vi "Comparison of BLAS and linear algebra VIs.vi"() -> ()   [LabVIEW 2023]
doc: "This example compares the use of the Basic Linear Algebra Subroutines (BLAS) VIs with the use of the Linear Algebra VIs."
uses:
  <vilib>/Analysis/BLAS.llb/LV_Transpose.ctl
  <vilib>/Analysis/baseanly.llb/Real Dot Product.vi
  <vilib>/Analysis/7linalg.llb/Complex Conjugate Transpose Matrix.vi
  <vilib>/Analysis/baseanly.llb/Complex A x Vector.vi
  <vilib>/Analysis/7linalg.llb/Real Transpose Matrix.vi
  <vilib>/Analysis/baseanly.llb/Real A x B.vi
  <vilib>/Analysis/2dsp.llb/Decimate (continuous, DBL).vi
  <vilib>/Analysis/BLAS.llb/zgemv - General Matrix-Vector Product (CDB).vi
  <vilib>/Analysis/Matrix/Numeric/Multiply/Multiply - R,RM.vi
  <vilib>/Analysis/Matrix/Numeric/Add/Add - RM,RM.vi
  <vilib>/Analysis/BLAS.llb/dgemm - General Matrix-Matrix Product (DBL).vi
  <vilib>/Analysis/NI_AALBLAS.lvlib
  <vilib>/Analysis/NI_AALBase.lvlib
  <vilib>/Analysis/Matrix/NI_Matrix.lvlib
  <vilib>/Analysis/NI_AALPro.lvlib
panel:
  in  "Tab Control":T1(tab)
  out "BLAS result":dbl
  in  "y":dbl[](array[numeric])=[4.0, 5.0, 6.0, 7.0, 8.0]
  in  "x":dbl[](array[numeric])=[1.0, 2.0, 3.0, 4.0, 5.0]
  in  "xInc":i32=2
  in  "yInc":i32=-2
  out "general linear algebra result":dbl
  out "BLAS result":cdb[](array[numeric])
  in  "y":cdb[](array[numeric])=[5.0+8.0i, 6.0+7.0i, 7.0+6.0i, 8.0+5.0i]
  in  "x":cdb[](array[numeric])=[1.0+3.0i, 2.0+5.0i, 3.0+7.0i]
  in  "A":cdb[][](array[numeric])=[[4.0+7.0i, 5.0+8.0i], [7.0+4.0i, 8.0+5.0i]]
  in  "operation A":T2=2 items=["Not Transposed", "Conjugated Transposed", "Transposed"]
  out "general linear algebra result":cdb[](array[numeric])
  in  "alpha":cdb=2.0+3.0i
  in  "beta":cdb=3.0+2.0i
  out "general linear algebra result":dbl[][](array[numeric])
  out "BLAS result":dbl[][](array[numeric])
  in  "C":dbl[][](array[numeric])=[[0.0, 0.0, 0.0], [0.0, 0.0, 0.0], [0.0, 0.0, 0.0]]
  in  "B":dbl[][](array[numeric])=[[5.0, 6.0, 7.0], [8.0, 9.0, 10.0], [11.0, 12.0, 13.0]]
  in  "A":dbl[][](array[numeric])=[[1.0, 0.0, 3.0], [0.0, 2.0, 0.0]]
  in  "operation A":T2 items=["Not Transposed", "Conjugated Transposed", "Transposed"]
  in  "operation B":T2 items=["Not Transposed", "Conjugated Transposed", "Transposed"]
  in  "alpha":dbl=2.0
  in  "beta":dbl=1.0
  # "Overview: This example compares the use of the Basic Linear Algebra Subroutines (BLAS) VIs with the use of the Linear Algebra VIs.\nRequirements: LabVIEW Full Development System\nInstructions: \n1. Run the VI.\n2. View the block diagram to see the difference between the BLAS VIs and the Linear Algebra VIs.\n3. Select a different tab and run the VI again to see a comparison of a different operation."
  # "Calculates the dot product of two real vectors."
  # "ddot = X . Y"
  # "Calculates the product of a general matrix and a vector."
  # "gemv=alpha*op(A)*X+beta*Y"
  # "Calculates the product of two general matrices."
  # "gemm=alpha*op(A)*op(B)+beta*C"
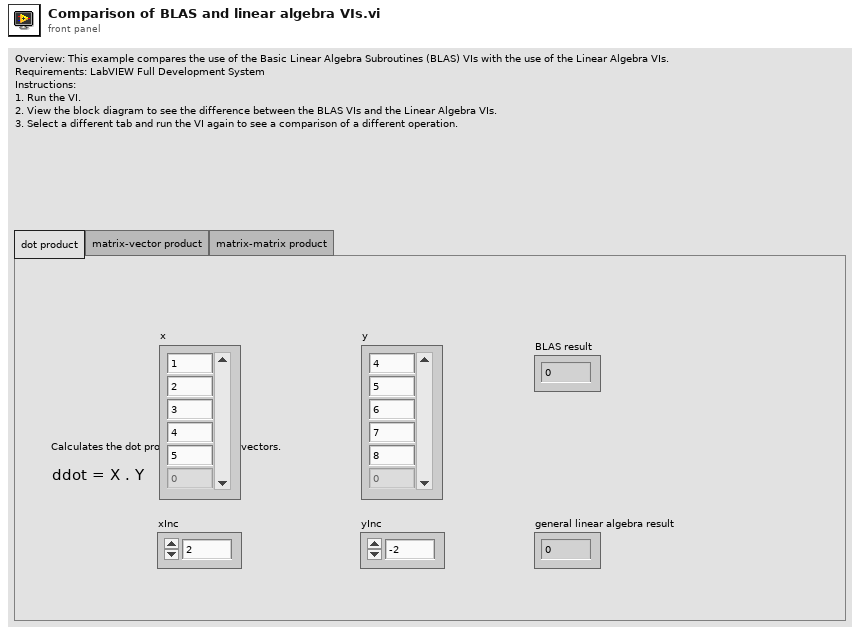
[diagram p1: front panel]
types:
  T1 = enum32{"dot product", "matrix-vector product", "matrix-matrix product"}
  T2 = typedef "NI_AALBLAS.lvlib/LV_Transpose.ctl" = i32
  T3 = typedef "NI_Matrix.lvlib/ComplexMatrix.ctl" = cdb[][]
  T4 = typedef "NI_Matrix.lvlib/RealMatrix.ctl" = dbl[][]
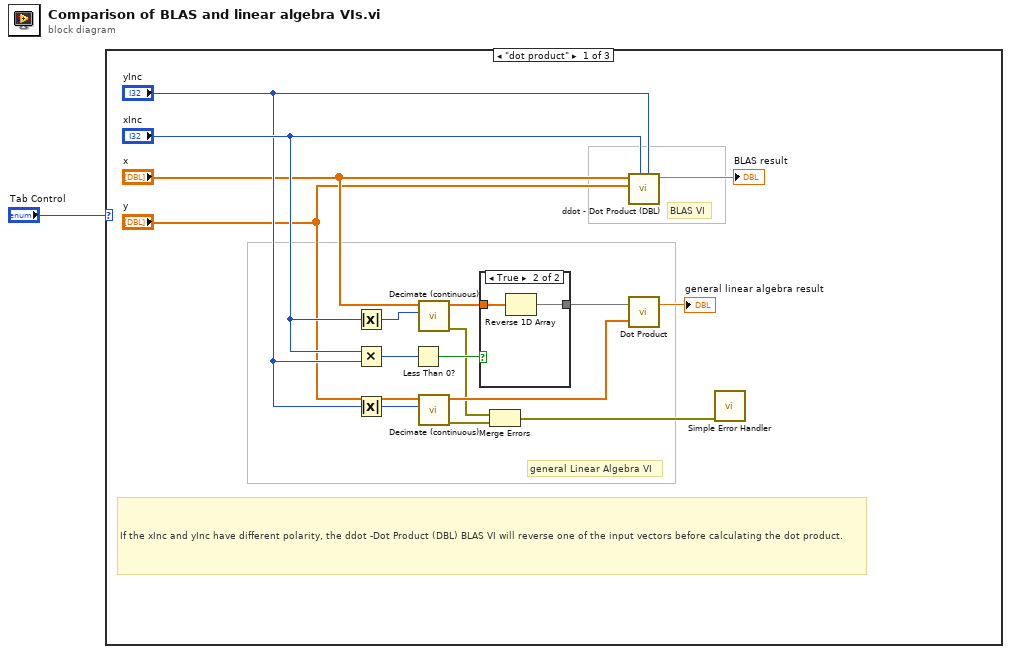
[diagram p0: block diagram]
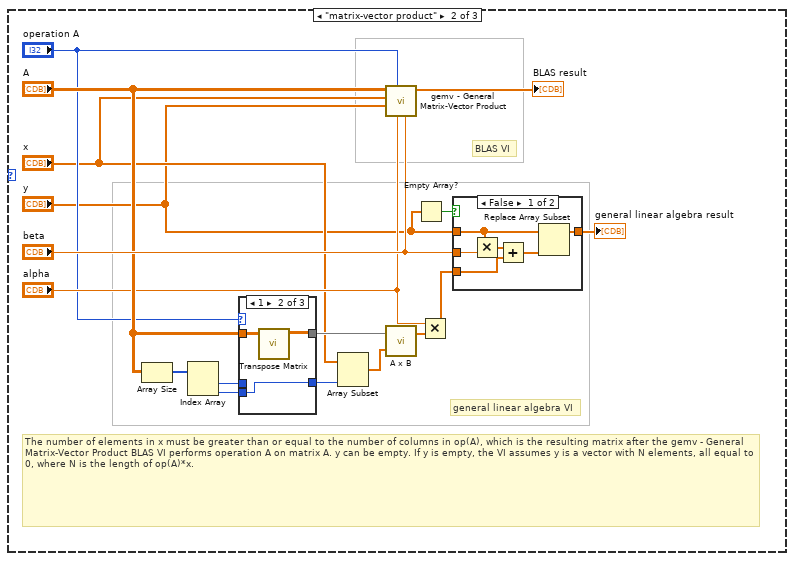
[diagram p3: hidden frame]
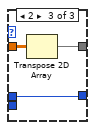
[diagram p6: hidden frame]
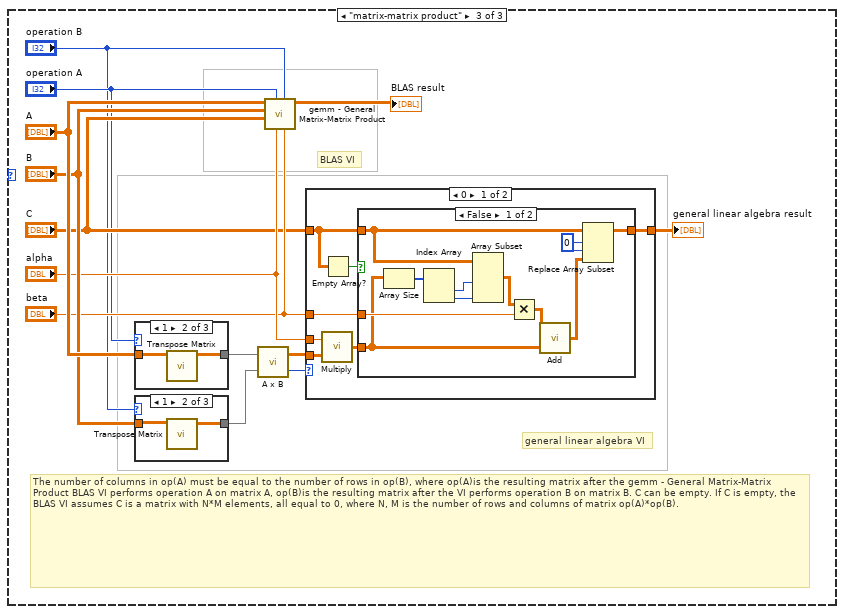
[diagram p7: hidden frame]
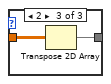
[diagram p11: hidden frame]
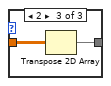
[diagram p13: hidden frame]
diagram:
  n1 = case shown="\"dot product\"" "Tab Control" {
    frame "dot product" {
      # "If the xInc and yInc have different polarity, the ddot -Dot Product (DBL) BLAS VI will reverse one of the input vectors before calculating the dot product."
      # "BLAS VI"
      # "general Linear Algebra VI"
      n2 = Absolute Value(x="xInc") -> (abs(x)=w9:i32)
      n3 = Multiply(x="xInc", y="yInc") -> (x*y=w14:i32)
      n4 = Absolute Value(x="yInc") -> (abs(x)=w8:i32)
      n5 = Less Than 0?(x=w14) -> (x < 0?=w13:bool)
      n6 = call-poly <vilib>:"Decimate (continuous).vi"("decimating factor"=w9, "X"="x") -> ("error out"=w3:errorcluster, "Decimated Array"=w5:dbl[])  [unwired: 4 in, 4 out]
      n7 = call-poly <vilib>:"Decimate (continuous).vi"("decimating factor"=w8, "X"="y") -> ("error out"=w4:errorcluster, "Decimated Array"=w6:dbl[])  [unwired: 4 in, 4 out]
      n8 = case shown="True" w13 {
        tunnel: w5 -> [w18 w20]
        tunnel: [w18 w19] -> w12
        frame False {
        }
        frame True {
          n9 = Reverse 1D Array(array=w20) -> (reversed array=w19:dbl[])
        }
      }
      n10 = Merge Errors(w3, w4) -> (w2:errorcluster)
      n11 = call <vilib>:"ddot - Dot Product (DBL).vi"("yInc"="yInc", "xInc"="xInc", "y"="y", "x"="x") -> ("ddot"=→"BLAS result":dbl)  [unwired: 7 out]
      n12 = call-poly <vilib>:"Dot Product.vi"("Y Vector"=w6, "X Vector"=w12) -> ("X * Y"=→"general linear algebra result":dbl)  [unwired: 1 out]
      n13 = call <vilib>:"Simple Error Handler.vi"("error in (no error)"=w2) -> ()  [unwired: 4 in, 5 out]
    }
    frame "matrix-vector product" {
      # "The number of elements in x must be greater than or equal to the number of columns in op(A), which is the resulting matrix after the gemv - General Matrix-Vector Product BLAS VI performs operation A on matrix A. y can be empty. If y is empty, the VI assumes y is a vector with N elements, all equal to 0, where N is the length of op(A)*x."
      # "BLAS VI"
      # "general linear algebra VI"
      n14 = Array Size(array="A") -> (size(s)=w31:i32[])
      n15 = Index Array(array=w31) -> (element #1=w28:i32, element #2=w27:i32)  [unwired: 2 in]
      n16 = case shown="1" "operation A" {
        tunnel: "A" -> [w46 w48 w52]
        tunnel: [w46 w47 w51] -> w34
        tunnel: w28 -> [w45 _ w50]
        tunnel: w27 -> [_ w49 _]
        tunnel: [w45 w49 w50] -> w26
        frame 0, Default {
        }
        frame 1 {
          n17 = call-poly <vilib>:"Transpose Matrix.vi"("Input Matrix"=w48) -> ("Matrix Conjugate Transpose"=w47:T3)  [unwired: 10 out]
        }
        frame 2 {
          n18 = Transpose 2D Array(2D array=w52) -> (transposed array=w51:cdb[][])
        }
      }
      n19 = Array Subset(array="x", length=w26) -> (w32:cdb[])  [unwired: 1 in]
      n20 = call-poly <vilib>:"gemv - General Matrix-Vector Product.vi"("beta"="beta", "alpha"="alpha", "operation A"="operation A", "y"="y", "x"="x", "A"="A") -> ("zgemv"=→"BLAS result":cdb[])  [unwired: 5 out]
      n21 = call-poly <vilib>:"A x B.vi"("Vector"=w32, "A"=w34) -> ("A x Vector"=w35:cdb[])  [unwired: 1 out]
      n22 = Empty Array?(array="y") -> (empty?=w23:bool)
      n23 = Multiply ("Multiply.vi")(x="alpha", y=w35) -> (x*y=w36:cdb[])
      n24 = case shown="False" w23 {
        tunnel: "beta" -> [w42 _]
        tunnel: "y" -> [w38 _]
        tunnel: w36 -> [w41 w44]
        tunnel: [w39 w44] -> w21
        frame False {
          n25 = Multiply(x=w38, y=w42) -> (x*y=w43:cdb[])
          n26 = Add(x=w43, y=w41) -> (x+y=w40:cdb[])
          n27 = Replace Array Subset(array=w38, new element=w40) -> (w39:cdb[])  [unwired: 1 in]
        }
        frame True {
        }
      }
      "general linear algebra result" <- w21
    }
    frame "matrix-matrix product" {
      # "The number of columns in op(A) must be equal to the number of rows in op(B), where op(A)is the resulting matrix after the gemm - General Matrix-Matrix Product BLAS VI performs operation A on matrix A, op(B)is the resulting matrix after the VI performs operation B on matrix B. C can be empty. If C is empty, the BLAS VI assumes C is a matrix with N*M elements, all equal to 0, where N, M is the number of rows and columns of matrix op(A)*op(B)."
      # "BLAS VI"
      # "general linear algebra VI"
      n28 = case shown="1" "operation A" {
        tunnel: "A" -> [w90 w92 w94]
        tunnel: [w90 w91 w93] -> w63
        frame 0, Default {
        }
        frame 1 {
          n29 = call-poly <vilib>:"Transpose Matrix.vi"("Input Matrix"=w92) -> ("Matrix Transpose"=w91:T4)  [unwired: 10 out]
        }
        frame 2 {
          n30 = Transpose 2D Array(2D array=w94) -> (transposed array=w93:dbl[][])
        }
      }
      n31 = case shown="1" "operation B" {
        tunnel: "B" -> [w85 w87 w89]
        tunnel: [w85 w86 w88] -> w61
        frame 0, Default {
        }
        frame 1 {
          n32 = call-poly <vilib>:"Transpose Matrix.vi"("Input Matrix"=w87) -> ("Matrix Transpose"=w86:T4)  [unwired: 10 out]
        }
        frame 2 {
          n33 = Transpose 2D Array(2D array=w89) -> (transposed array=w88:dbl[][])
        }
      }
      n34 = call-poly <vilib>:"A x B.vi"("B"=w61, "A"=w63) -> ("error"=w55:i32, "A x B"=w56:T4)
      n35 = call-poly <vilib>:"gemm - General Matrix-Matrix Product.vi"("beta"="beta", "operation B"="operation B", "alpha"="alpha", "operation A"="operation A", "C"="C", "B"="B", "A"="A") -> ("dgemm"=→"BLAS result":T4)  [unwired: 4 out]
      n36 = case shown="0" w55 {
        tunnel: "alpha" -> [w67 _]
        tunnel: "beta" -> [w72 _]
        tunnel: [w71 _] -> w58
        tunnel: "C" -> [w70 _]
        tunnel: w56 -> [w66 _]
        frame 0 {
          n37 = call-poly <vilib>:"Multiply.vi"("Real Matrix A"=w66, "Real Scalar c"=w67) -> ("c * A"=w68:T4)
          n38 = Empty Array?(array=w70) -> (empty?=w69:bool)
          n39 = case shown="False" w69 {
            tunnel: w72 -> [w83 _]
            tunnel: [w80 w84] -> w71
            tunnel: w70 -> [w78 _]
            tunnel: w68 -> [w73 w84]
            frame False {
              w81 = 0 ("index (row)")
              n40 = Array Size(array=w73) -> (size(s)=w76:i32[])
              n41 = Index Array(array=w76) -> (element #1=w75:i32, element #2=w74:i32)  [unwired: 2 in]
              n42 = Array Subset(array=w78, length (row)=w75, length (col)=w74) -> (w77:dbl[][])  [unwired: 2 in]
              n43 = Multiply ("Multiply.vi")(x=w77, y=w83) -> (x*y=w79:dbl[][])
              n44 = call-poly <vilib>:"Add.vi"("Real Matrix B"=w73, "Real Matrix A"=w79) -> ("A + B"=w82:T4)
              n45 = Replace Array Subset(array=w78, new element=w82, index (row)=w81, index (col)=w81) -> (w80:dbl[][])
            }
            frame True {
            }
          }
        }
        frame Default {
        }
      }
      "general linear algebra result" <- w58
    }
  }
